vi "Read_From_File.vi"   [LabVIEW 2018]
uses:
  Global_Variables/Dashboard_Globals.vi
  <vilib>/Rock Robotics/Network Tables/NT Write Number.vi
types:
  T1 = enum16{"open", "replace", "create", "open or create", "replace or create", "replace or create with confirmation"}
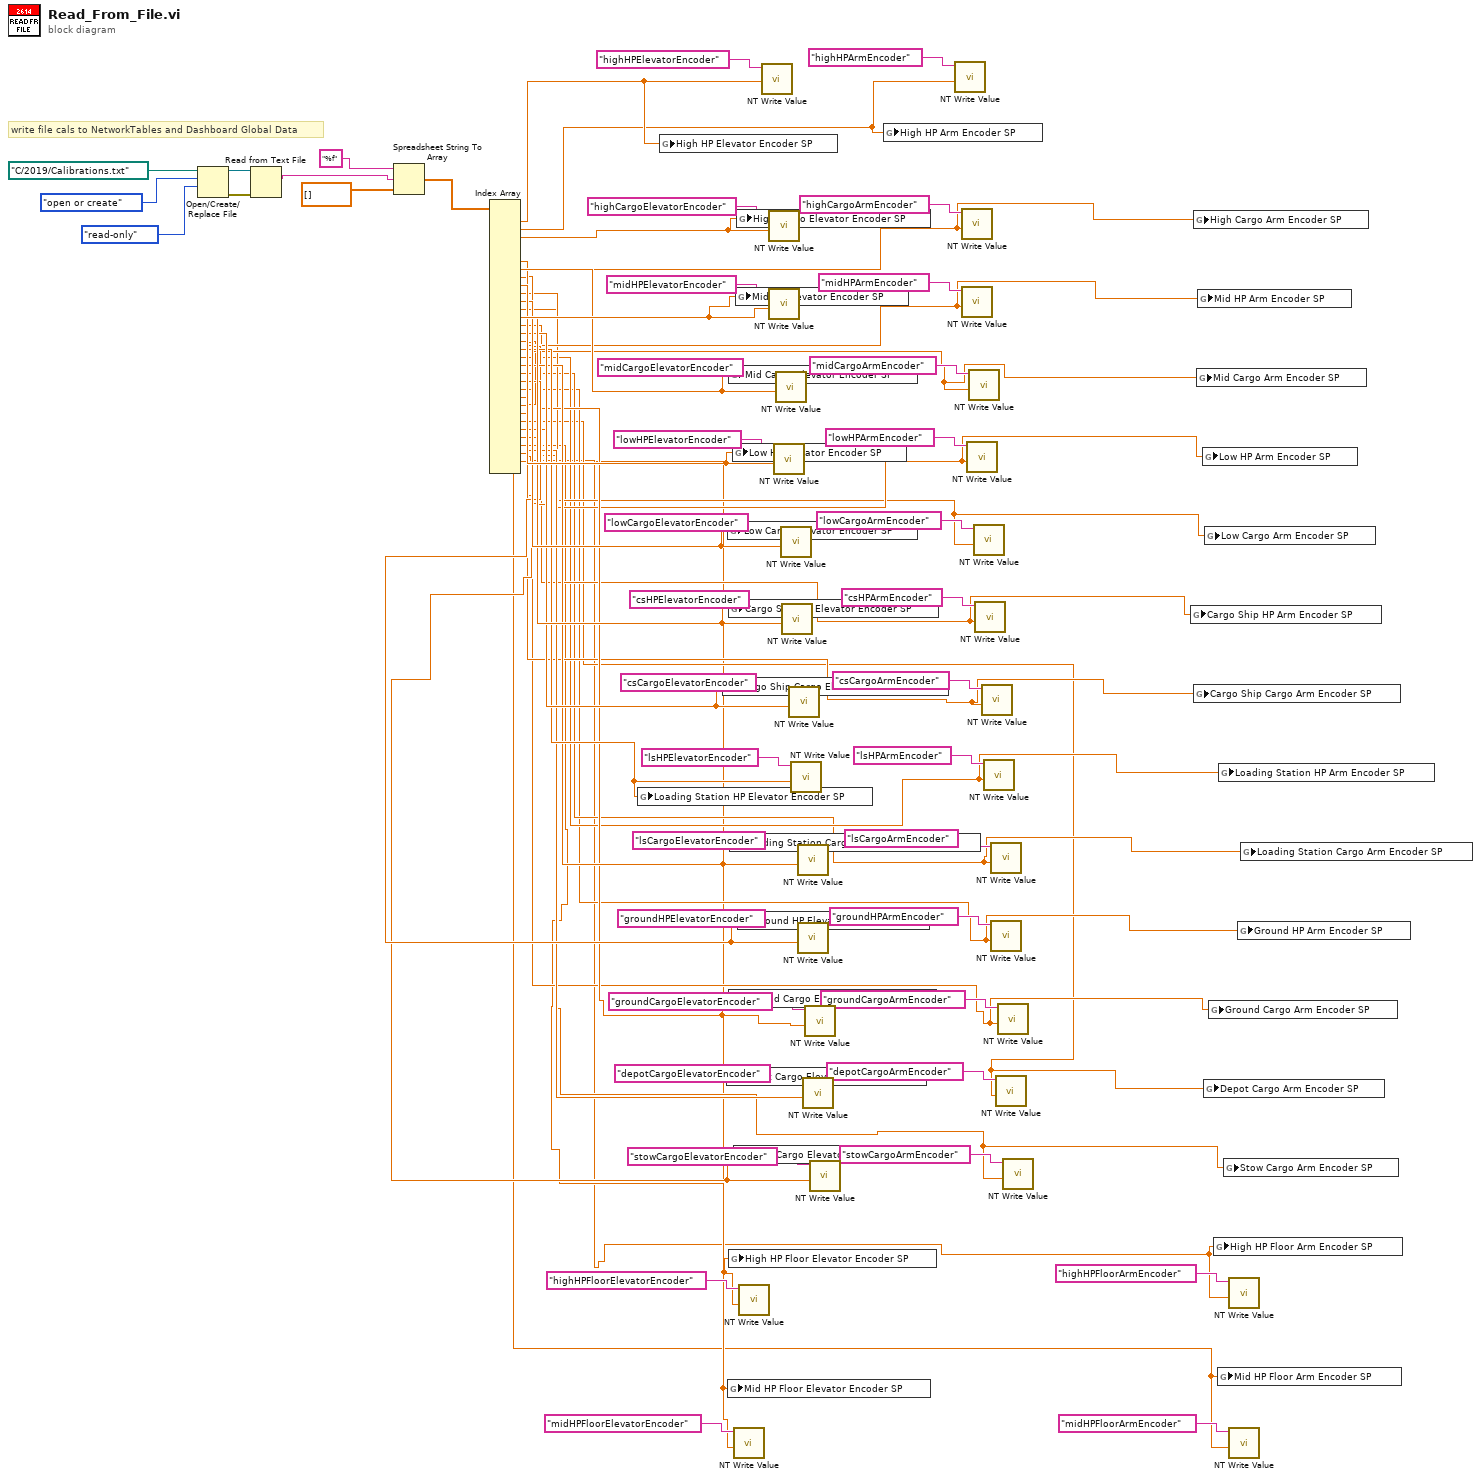
[diagram p0: block diagram]
diagram:
  # "write file cals to NetworkTables and Dashboard Global Data"
  n1 = Open/Create/Replace File(file path (use dialog)=path "C:/2019/Calibrations.txt" ("file (use dialog)"), operation (0:open)=T1."open or create", access (0:read/write)=enum16{"read/write", "read-only", "write-only"}."read-only") -> (refnum out=w45:refnum<file>, error out=w44:errorcluster)  [unwired: 3 in, 1 out]
  n2 = Read from Text File(file (use dialog)=w45, error in=w44) -> (text=w38:string)  [unwired: 2 in, 3 out]
  n3 = Spreadsheet String To Array(format string="%f", spreadsheet string=w38, array type (2D Dbl)=dbl[] []) -> (array=w37:dbl[])  [unwired: 1 in]
  n4 = Index Array(array=w37) -> (element #1=w36:dbl, element #2=w22:dbl, element #3=w35:dbl, element #4=w21:dbl, element #5=w34:dbl, element #6=w20:dbl, element #7=w33:dbl, element #8=w19:dbl, element #9=w32:dbl, element #10=w18:dbl, element #11=w31:dbl, element #12=w17:dbl, element #13=w30:dbl, element #14=w16:dbl, element #15=w29:dbl, element #16=w15:dbl, element #17=w28:dbl, element #18=w14:dbl, element #19=w27:dbl, element #20=w13:dbl, element #21=w26:dbl, element #22=w12:dbl, element #23=w25:dbl, element #24=w11:dbl, element #25=w24:dbl, element #26=w10:dbl, element #27=w23:dbl, element #28=w9:dbl, element #29=w4:dbl, element #30=w3:dbl, element #31=w2:dbl, element #32=w1:dbl)  [unwired: 32 in]
  n5 = global write "Dashboard_Globals.vi" "Loading Station HP Elevator Encoder SP"(w28) -> ()
  n6 = global write "Dashboard_Globals.vi" "High HP Elevator Encoder SP"(w36) -> ()
  n7 = global write "Dashboard_Globals.vi" "Cargo Ship Cargo Elevator Encoder SP"(w29) -> ()
  n8 = global write "Dashboard_Globals.vi" "Depot Cargo Elevator Encoder SP"(w24) -> ()
  n9 = global write "Dashboard_Globals.vi" "Low Cargo Elevator Encoder SP"(w31) -> ()
  n10 = global write "Dashboard_Globals.vi" "Mid HP Floor Elevator Encoder SP"(w2) -> ()
  n11 = global write "Dashboard_Globals.vi" "Mid Cargo Elevator Encoder SP"(w33) -> ()
  n12 = global write "Dashboard_Globals.vi" "Cargo Ship HP Elevator Encoder SP"(w30) -> ()
  n13 = global write "Dashboard_Globals.vi" "Ground Cargo Elevator Encoder SP"(w25) -> ()
  n14 = global write "Dashboard_Globals.vi" "High HP Floor Elevator Encoder SP"(w4) -> ()
  n15 = global write "Dashboard_Globals.vi" "Loading Station Cargo Elevator Encoder SP"(w27) -> ()
  n16 = global write "Dashboard_Globals.vi" "Low HP Elevator Encoder SP"(w32) -> ()
  n17 = global write "Dashboard_Globals.vi" "Stow Cargo Elevator Encoder SP"(w23) -> ()
  n18 = call-poly <vilib>:"NT Write Value.vi"("Numeric"=w2, "Name"="midHPFloorElevatorEncoder") -> ()  [unwired: 9 in, 1 out]
  n19 = global write "Dashboard_Globals.vi" "Mid HP Elevator Encoder SP"(w34) -> ()
  n20 = global write "Dashboard_Globals.vi" "High Cargo Elevator Encoder SP"(w35) -> ()
  n21 = global write "Dashboard_Globals.vi" "Ground HP Elevator Encoder SP"(w26) -> ()
  n22 = call-poly <vilib>:"NT Write Value.vi"("Numeric"=w4, "Name"="highHPFloorElevatorEncoder") -> ()  [unwired: 9 in, 1 out]
  n23 = call-poly <vilib>:"NT Write Value.vi"("Numeric"=w36, "Name"="highHPElevatorEncoder") -> ()  [unwired: 9 in, 1 out]
  n24 = call-poly <vilib>:"NT Write Value.vi"("Numeric"=w35, "Name"="highCargoElevatorEncoder") -> ()  [unwired: 9 in, 1 out]
  n25 = call-poly <vilib>:"NT Write Value.vi"("Numeric"=w34, "Name"="midHPElevatorEncoder") -> ()  [unwired: 9 in, 1 out]
  n26 = call-poly <vilib>:"NT Write Value.vi"("Numeric"=w32, "Name"="lowHPElevatorEncoder") -> ()  [unwired: 9 in, 1 out]
  n27 = call-poly <vilib>:"NT Write Value.vi"("Numeric"=w33, "Name"="midCargoElevatorEncoder") -> ()  [unwired: 9 in, 1 out]
  n28 = call-poly <vilib>:"NT Write Value.vi"("Numeric"=w31, "Name"="lowCargoElevatorEncoder") -> ()  [unwired: 9 in, 1 out]
  n29 = call-poly <vilib>:"NT Write Value.vi"("Numeric"=w30, "Name"="csHPElevatorEncoder") -> ()  [unwired: 9 in, 1 out]
  n30 = call-poly <vilib>:"NT Write Value.vi"("Numeric"=w29, "Name"="csCargoElevatorEncoder") -> ()  [unwired: 9 in, 1 out]
  n31 = call-poly <vilib>:"NT Write Value.vi"("Numeric"=w28, "Name"="lsHPElevatorEncoder") -> ()  [unwired: 9 in, 1 out]
  n32 = call-poly <vilib>:"NT Write Value.vi"("Numeric"=w27, "Name"="lsCargoElevatorEncoder") -> ()  [unwired: 9 in, 1 out]
  n33 = call-poly <vilib>:"NT Write Value.vi"("Numeric"=w26, "Name"="groundHPElevatorEncoder") -> ()  [unwired: 9 in, 1 out]
  n34 = call-poly <vilib>:"NT Write Value.vi"("Numeric"=w24, "Name"="depotCargoElevatorEncoder") -> ()  [unwired: 9 in, 1 out]
  n35 = call-poly <vilib>:"NT Write Value.vi"("Numeric"=w25, "Name"="groundCargoElevatorEncoder") -> ()  [unwired: 9 in, 1 out]
  n36 = call-poly <vilib>:"NT Write Value.vi"("Numeric"=w23, "Name"="stowCargoElevatorEncoder") -> ()  [unwired: 9 in, 1 out]
  n37 = global write "Dashboard_Globals.vi" "High HP Arm Encoder SP"(w22) -> ()
  n38 = call-poly <vilib>:"NT Write Value.vi"("Numeric"=w22, "Name"="highHPArmEncoder") -> ()  [unwired: 9 in, 1 out]
  n39 = call-poly <vilib>:"NT Write Value.vi"("Numeric"=w21, "Name"="highCargoArmEncoder") -> ()  [unwired: 9 in, 1 out]
  n40 = call-poly <vilib>:"NT Write Value.vi"("Numeric"=w20, "Name"="midHPArmEncoder") -> ()  [unwired: 9 in, 1 out]
  n41 = call-poly <vilib>:"NT Write Value.vi"("Numeric"=w18, "Name"="lowHPArmEncoder") -> ()  [unwired: 9 in, 1 out]
  n42 = call-poly <vilib>:"NT Write Value.vi"("Numeric"=w19, "Name"="midCargoArmEncoder") -> ()  [unwired: 9 in, 1 out]
  n43 = call-poly <vilib>:"NT Write Value.vi"("Numeric"=w17, "Name"="lowCargoArmEncoder") -> ()  [unwired: 9 in, 1 out]
  n44 = call-poly <vilib>:"NT Write Value.vi"("Numeric"=w16, "Name"="csHPArmEncoder") -> ()  [unwired: 9 in, 1 out]
  n45 = call-poly <vilib>:"NT Write Value.vi"("Numeric"=w15, "Name"="csCargoArmEncoder") -> ()  [unwired: 9 in, 1 out]
  n46 = call-poly <vilib>:"NT Write Value.vi"("Numeric"=w14, "Name"="lsHPArmEncoder") -> ()  [unwired: 9 in, 1 out]
  n47 = call-poly <vilib>:"NT Write Value.vi"("Numeric"=w13, "Name"="lsCargoArmEncoder") -> ()  [unwired: 9 in, 1 out]
  n48 = call-poly <vilib>:"NT Write Value.vi"("Numeric"=w12, "Name"="groundHPArmEncoder") -> ()  [unwired: 9 in, 1 out]
  n49 = call-poly <vilib>:"NT Write Value.vi"("Numeric"=w10, "Name"="depotCargoArmEncoder") -> ()  [unwired: 9 in, 1 out]
  n50 = call-poly <vilib>:"NT Write Value.vi"("Numeric"=w11, "Name"="groundCargoArmEncoder") -> ()  [unwired: 9 in, 1 out]
  n51 = call-poly <vilib>:"NT Write Value.vi"("Numeric"=w9, "Name"="stowCargoArmEncoder") -> ()  [unwired: 9 in, 1 out]
  n52 = global write "Dashboard_Globals.vi" "Cargo Ship HP Arm Encoder SP"(w16) -> ()
  n53 = global write "Dashboard_Globals.vi" "High Cargo Arm Encoder SP"(w21) -> ()
  n54 = global write "Dashboard_Globals.vi" "Cargo Ship Cargo Arm Encoder SP"(w15) -> ()
  n55 = global write "Dashboard_Globals.vi" "Mid Cargo Arm Encoder SP"(w19) -> ()
  n56 = global write "Dashboard_Globals.vi" "Mid HP Arm Encoder SP"(w20) -> ()
  n57 = global write "Dashboard_Globals.vi" "Low HP Arm Encoder SP"(w18) -> ()
  n58 = global write "Dashboard_Globals.vi" "Depot Cargo Arm Encoder SP"(w10) -> ()
  n59 = global write "Dashboard_Globals.vi" "Low Cargo Arm Encoder SP"(w17) -> ()
  n60 = global write "Dashboard_Globals.vi" "Ground Cargo Arm Encoder SP"(w11) -> ()
  n61 = global write "Dashboard_Globals.vi" "High HP Floor Arm Encoder SP"(w3) -> ()
  n62 = global write "Dashboard_Globals.vi" "Mid HP Floor Arm Encoder SP"(w1) -> ()
  n63 = global write "Dashboard_Globals.vi" "Loading Station HP Arm Encoder SP"(w14) -> ()
  n64 = global write "Dashboard_Globals.vi" "Stow Cargo Arm Encoder SP"(w9) -> ()
  n65 = call-poly <vilib>:"NT Write Value.vi"("Numeric"=w3, "Name"="highHPFloorArmEncoder") -> ()  [unwired: 9 in, 1 out]
  n66 = call-poly <vilib>:"NT Write Value.vi"("Numeric"=w1, "Name"="midHPFloorArmEncoder") -> ()  [unwired: 9 in, 1 out]
  n67 = global write "Dashboard_Globals.vi" "Ground HP Arm Encoder SP"(w12) -> ()
  n68 = global write "Dashboard_Globals.vi" "Loading Station Cargo Arm Encoder SP"(w13) -> ()
